vi "Read CSM Status By CSM.vi"(6 "Config Path":path, 8 "Error In":errorcluster caption="Error in (no error)", 11 "CSM Name":string) -> (0 "Error Out":errorcluster, 3 "Array 3":cluster{"Status":string, "InState":string}[](array[cluster]))   [LabVIEW 2017, in "CSM-Helper API with lvcsm Support.lvlib"]
uses:
  CSM-Helper API with lvcsm Support.lvlib
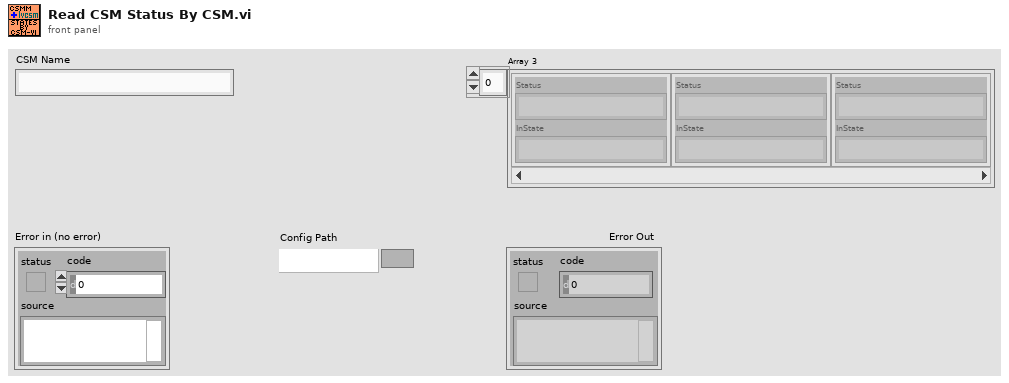
[diagram p1: front panel]
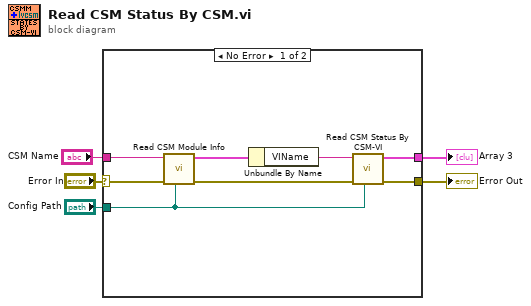
[diagram p0: block diagram]
diagram:
  n1 = case shown="No Error" "Error In" {
    selector: "Error In" -> [w13 w14]
    tunnel: [w11 w14] -> w4
    tunnel: "Config Path" -> [w8 _]
    tunnel: "CSM Name" -> [w7 _]
    tunnel: [w9 _] -> w1
    frame No Error {
      n2 = call "Read CSM Module Info.vi"("Config Path"=w8, "error in (no error)"=w13, "CSM Name"=w7) -> ("error out"=w12:errorcluster, "Cluster"=w10:cluster{"VIName":string})  [unwired: 7 in]
      n3 = Unbundle By Name(w10) -> ("VIName"=w6:string)
      n4 = call "Read CSM Status By CSM-VI.vi"("Config Path"=w8, "Error In"=w12, "CSM VI"=w6) -> ("Error Out"=w11:errorcluster, "Array 3"=w9:cluster{"Status":string, "InState":string}[])  [unwired: 7 in]
    }
    frame Error {
    }
  }
  "Error Out" <- w4
  "Array 3" <- w1
